vi "DelayLineMove.vi"(1 "Points":cluster{string, "data":u64, "data":dbl}, 2 "Inst_param":T1) -> ()   [LabVIEW 2013]
uses:
  Drivers/Set Parameter.ctl
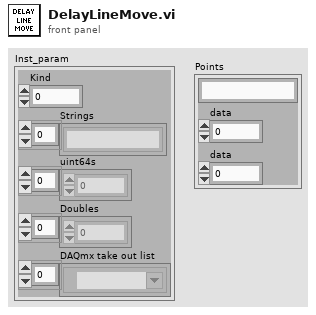
[diagram p1: front panel]
types:
  T1 = cluster{"Kind":u16, "Strings":string[], "uint64s":u64[], "Doubles":dbl[], "DAQmx take out list":refnum<k21>[]}
  T2 = typedef "Set Parameter.ctl" = enum16{"Acceleration (A)", "Baud Rate (BD)", "Counter 1 (C1)", "Counter 2 (C2)", "Control C Software Reset (CE)", "Check Sum Enable (CK)", "Clock Mode (CM)", "Clock Mode Ratio (CR)", "Clock Mode Out Step Width (CW)", "Deceleration (D)", "Digital Filtering, Input 1 (D1)", "Digital Filtering, Input 2 (D2)", "Digital Filtering, Input 3 (D3)", "Digital Filtering, Input 4 (D4)", "Digital Filtering, Input 5 (D5)", "Digital Filtering, Input 9 (D9)", "Digital Filtering, Input 10 (D10)", "Digital Filtering, Input 11 (D11)", "Digital Filtering, Input 12 (D12)", "Deadband (DB)", "Decrement Variable (DC)", "Enable/Disable Drive (DE)", "Device Name (DN)", "End Program Execution (E)", "Encoder Function Enable (EE)", "Encoder Lines (EL)", "Echo Mode (EM)", "Escape (ES)", "Execute Program at Address (EX)", "Hold (H)", "Hold Current (HC)", "Hold Current Delay Time (HI)", "Home to Encoder Index (HM)", "Home to Home Switch (HT)", "Increment Variable (IC)", "Initialize Parameters to NVM (IP)", "Input into Variable (IV)", "Jog Enable (JE)", "Limit Stop Mode (LM)", "Move Absolute (MA)", "Move Relative (MR)", "MicroStepping Select (MS)", "Motor Settling Delay Time (MT)", "Output 1 (O1)", "Output 2 (O2)", "Output 3 (O3)", "Output 4 (O4)", "Output 9 (O9)", "Output 10 (O10)", "Output 11 (O11)", "Output 12 (O12)", "Output High Byte (9-12) (OH)", "Output Low Byte (1-4) (OL)", "Output Total (1-4 and 9-12) (OT)", "Position Maintenance (PM)", "Party Mode (PY)", "Register 1 (R1)", "Register 2 (R2)", "Register 3 (R3)", "Register 4 (R4)", "Run Current (RC)", "Stall Factor (SF)", "Slew (SL)", "Stall Mode Set (SM)", "Upgrade Firmware (UG)", "Velocity Initial (VI)", "Velocity Maximum (VM)"}
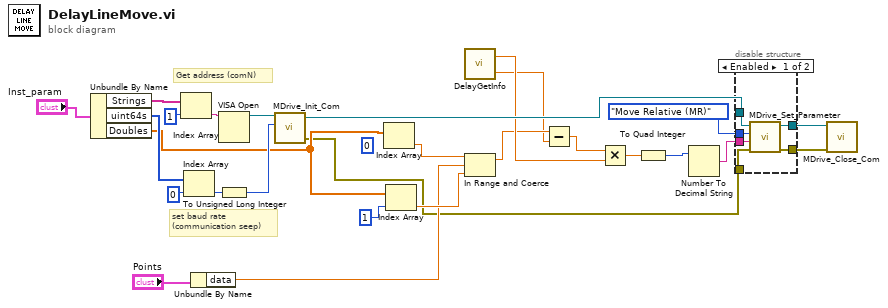
[diagram p0: block diagram]
diagram:
  (unwired) 0
  # "Get address (comN)"
  # "set baud rate\n(communication seep)"
  n1 = Unbundle By Name("Inst_param") -> ("Strings"=w27:string[], "uint64s"=w20:u64[], "Doubles"=w17:dbl[])
  n2 = Index Array(array=w27, index=1) -> (element=w25:string)
  n3 = Index Array(array=w20, index=0) -> (element=w22:u64)
  n4 = Unbundle By Name("Points") -> ("data"=w13:dbl)
  n5 = VISA Open(VISA resource name=w25) -> (VISA resource name=w24:refnum<visa-resource-name>)  [unwired: 4 in, 1 out]
  n6 = To Unsigned Long Integer(number=w22) -> (unsigned 32bit integer=w21:u32)
  n7 = call "MDrive_Init_Com.vi"("VISA resource name"=w24, "baud rate"=w21) -> ("VISA resource name out"=w8:refnum<visa-resource-name>, "error out"=w5:errorcluster)  [unwired: 5 in]
  n8 = Index Array(array=w17) -> (element=w15:dbl)  [unwired: 1 in]
  n9 = Index Array(array=w17, index=1) -> (element=w16:dbl)
  n10 = call "DelayGetInfo.vi"() -> ("Delay position (ps)"=w2:dbl, "Conversion"=w4:dbl)  [unwired: 2 in]
  n11 = In Range and Coerce(upper limit=w15, x=w13, lower limit=w16) -> (coerced(x)=w3:dbl)  [unwired: 1 out]
  n12 = Subtract(x=w3, y=w2) -> (x-y=w12:dbl)
  n13 = Multiply(x=w12, y=w4) -> (x*y=w9:dbl)
  n14 = To Quad Integer(1:w9) -> (0:w1:i64)
  n15 = Number To Decimal String(number=w1) -> (decimal integer string=w10:string)  [unwired: 1 in]
  n16 = disable-structure shown="Enabled" {
    disable-tunnel: Set_Parameter."Move Relative (MR)" ("Set Parameter") -> [w33 _]
    disable-tunnel: w10 -> [w32 _]
    disable-tunnel: w8 -> [w31 w35]
    disable-tunnel: [w30 w35] -> w7
    disable-tunnel: [w29 w34] -> w6
    disable-tunnel: w5 -> [w28 w34]
    frame Enabled {
      n17 = call "MDrive_Set_Parameter.vi"("error out 2"=w28, "Parameter Setpoint"=w32, "Set Parameter"=w33, "VISA resource name out 2"=w31) -> ("error out"=w29:errorcluster, "VISA resource name out"=w30:refnum<visa-resource-name>)  [unwired: 1 in, 1 out]
    }
    frame Disabled {
    }
  }
  n18 = call "MDrive_Close_Com.vi"("error out"=w6, "VISA resource name out"=w7) -> ()  [unwired: 2 in]
